vi "invisible button responseAI.vi"() -> (8 "desired move":bool[][](array[boolean]), 15 "stop loop":bool)   [LabVIEW 2019]
doc: "This subvi generates a 3x3 desired move boolean array based upon the Smart AI totally not Random\nJuan Gamez\nP3600\nCSUSB Physics"
uses:
  <vilib>/numeric/Random Number (Range) U64.vi
  <vilib>/numeric/sub_Random U32.vi
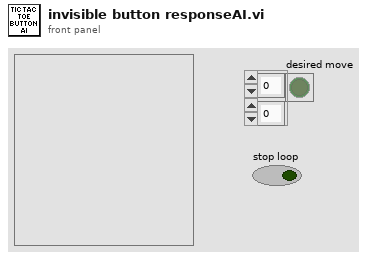
[diagram p1: front panel]
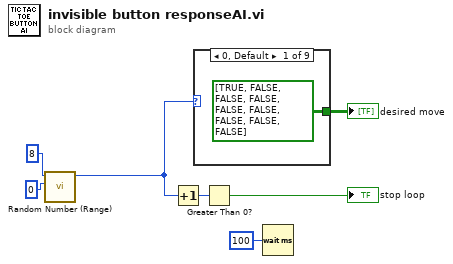
[diagram p0: block diagram]
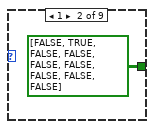
[diagram p2: hidden frame]
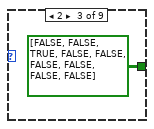
[diagram p3: hidden frame]
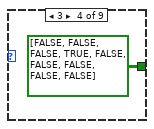
[diagram p4: hidden frame]
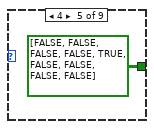
[diagram p5: hidden frame]
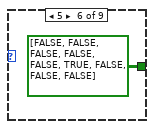
[diagram p6: hidden frame]
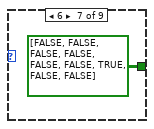
[diagram p7: hidden frame]
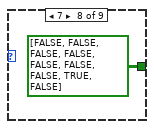
[diagram p8: hidden frame]
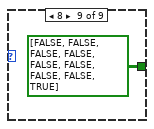
[diagram p9: hidden frame]
diagram:
  n1 = call-poly <vilib>:"Random Number (Range).vi"("lower bound (0)"=u64 0, "upper bound (100)"=u64 8) -> ("number"=w2:u64)  [unwired: 9 in]
  n2 = Increment(x=w2) -> (x+1=w5:u64)
  n3 = case shown="0, Default" w2 {
    tunnel: [bool[][] [[TRUE, FALSE, FALSE], [FALSE, FALSE, FALSE], [FALSE, FALSE, FALSE]] ("desired move") bool[][] [[FALSE, TRUE, FALSE], [FALSE, FALSE, FALSE], [FALSE, FALSE, FALSE]] ("desired move") bool[][] [[FALSE, FALSE, TRUE], [FALSE, FALSE, FALSE], [FALSE, FALSE, FALSE]] ("desired move") bool[][] [[FALSE, FALSE, FALSE], [TRUE, FALSE, FALSE], [FALSE, FALSE, FALSE]] ("desired move") bool[][] [[FALSE, FALSE, FALSE], [FALSE, TRUE, FALSE], [FALSE, FALSE, FALSE]] ("desired move") bool[][] [[FALSE, FALSE, FALSE], [FALSE, FALSE, TRUE], [FALSE, FALSE, FALSE]] ("desired move") bool[][] [[FALSE, FALSE, FALSE], [FALSE, FALSE, FALSE], [TRUE, FALSE, FALSE]] ("desired move") bool[][] [[FALSE, FALSE, FALSE], [FALSE, FALSE, FALSE], [FALSE, TRUE, FALSE]] ("desired move") bool[][] [[FALSE, FALSE, FALSE], [FALSE, FALSE, FALSE], [FALSE, FALSE, TRUE]] ("desired move")] -> w7
    frame 0, Default {
    }
    frame 1 {
    }
    frame 2 {
    }
    frame 3 {
    }
    frame 4 {
    }
    frame 5 {
    }
    frame 6 {
    }
    frame 7 {
    }
    frame 8 {
    }
  }
  "desired move" <- w7
  n4 = Greater Than 0?(x=w5) -> (x > 0?=→"stop loop":bool)
  n5 = Wait (ms)(milliseconds to wait=u32 100) -> ()  [unwired: 1 out]
